vi "set board and channels.vi"(10 "channels in":string[](array[string])=["0"], 11 "device in":i16=1) -> (0 "failed":bool, 1 "Canceled":bool, 2 "channels out":string[](array[string])=["0"], 3 "device out":i16=1)   [LabVIEW 2010]
panel:
  in  "Cancel":bool
  in  "OK":bool
  in  "channels":string[](array[string])=["0:5"]
  in  "device":i16=1
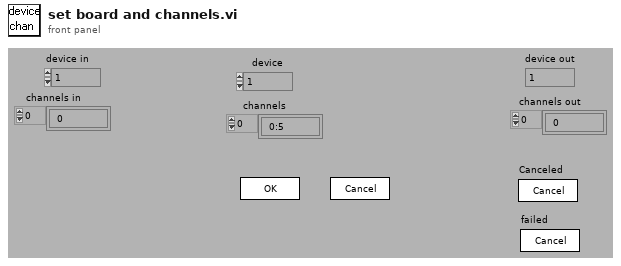
[diagram p1: front panel]
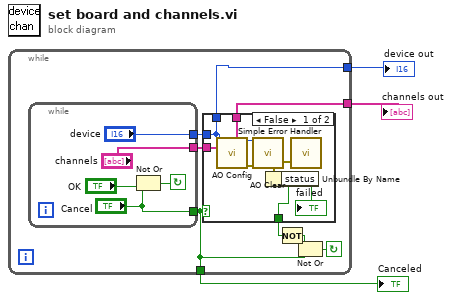
[diagram p0: block diagram]
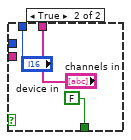
[diagram p2: hidden frame]
diagram:
  n1 = while {
    tunnel: [w4] -> w1
    tunnel: [w5] -> w2
    tunnel: [w10] -> w3
    stop <- w11 continue-if-true
    n2 = while {
      tunnel: ["Cancel"] -> w10
      tunnel: ["channels"] -> w7
      tunnel: ["device"] -> w6
      stop <- w14 continue-if-true
      n3 = Not Or(1:"Cancel", 2:"OK") -> (0:w14:bool)
    }
    n4 = case shown="False" w10 {
      tunnel: w6 -> [w18 _]
      tunnel: w7 -> [w17 _]
      tunnel: [w19 FALSE ("status")] -> w8
      tunnel: [w18 "device in"] -> w5
      tunnel: [w17 "channels in"] -> w4
      frame False {
        n5 = call "AO Config.vi"("device (1)"=w18, "channels (0)"=w17) -> ("taskID"=w21:u32, "error out"=w22:errorcluster)  [unwired: 11 in, 1 out]
        n6 = call "AO Clear.vi"("error in (no error)"=w22, "taskID in"=w21) -> ("error out"=w20:errorcluster)  [unwired: 4 in, 1 out]
        n7 = Unbundle By Name(w20) -> ("status"=w19:bool)
        "failed" <- w19
        n8 = call <vilib>:"Simple Error Handler.vi"("error in (no error)"=w20) -> ()  [unwired: 4 in, 5 out]
      }
      frame True {
      }
    }
    n9 = Not(x=w8) -> (.not. x?=w9:bool)
    n10 = Not Or(1:w10, 2:w9) -> (0:w11:bool)
  }
  "device out" <- w2
  "channels out" <- w1
  "Canceled" <- w3
